vi "Switch Box Signal Select Control.vi"(0 "PhyChls":tag="Dev1/port0/line1:2", 1 "line grouping":i32(ring) items=["one channel for each line", "one channel for all lines"], 2 "Signal":T1(ring), 5 "All OFF":bool, 7 "Dout Inv":bool[](array[boolean])=[FALSE, FALSE], 11 "ErrIn":errorcluster, 12 "SimOn":bool, 13 "Init":bool, 14 "Stop":bool) -> (15 "ErrOut":errorcluster)   [LabVIEW 2013]
uses:
  <vilib>/DAQmx/write.llb/DAQmx Write (Digital 1D Bool NChan 1Samp 1Line).vi
  <vilib>/DAQmx/create/channels.llb/DAQmx Create Channel (DO-Digital Output).vi
  <vilib>/DAQmx/miscellaneous.llb/DAQmx Fill In Error Info.vi
panel:
  # "ER2007"
  # "SCL1 -> SCL2"
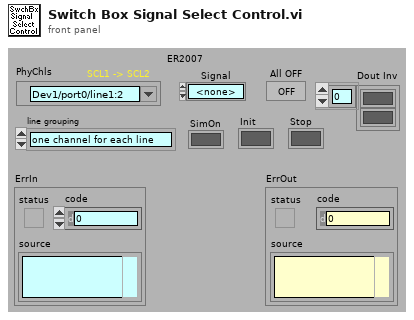
[diagram p1: front panel]
types:
  T1 = enum16{"<none>", "Signal 1", "Signal 2", "Signal 3"}
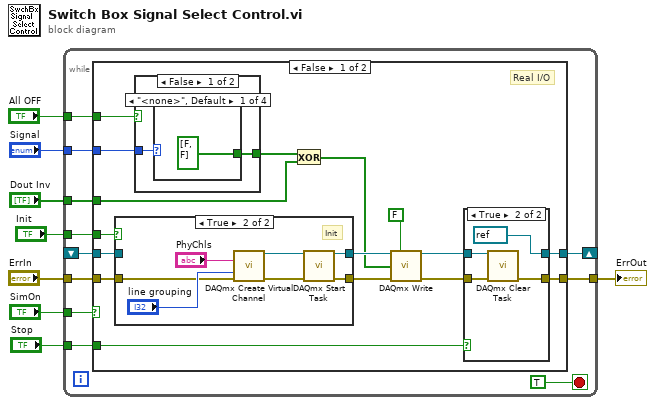
[diagram p0: block diagram]
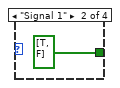
[diagram p4: hidden frame]
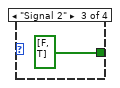
[diagram p5: hidden frame]
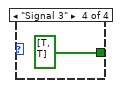
[diagram p6: hidden frame]
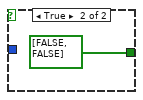
[diagram p7: hidden frame]
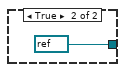
[diagram p9: hidden frame]
diagram:
  n1 = while {
    tunnel: "ErrIn" -> [w19]
    tunnel: [w18] -> w7
    tunnel: "SimOn" -> [w17]
    tunnel: "Stop" -> [w16]
    tunnel: "All OFF" -> [w15]
    tunnel: "Signal" -> [w14]
    tunnel: "Dout Inv" -> [w13]
    shift-right: [w12] -> _
    shift-left: _ -> [w10]
    tunnel: "Init" -> [w9]
    stop <- TRUE stop-if-true
    n2 = case shown="False" w17 {
      tunnel: w19 -> [w35 w61]
      tunnel: [w29 w61] -> w18
      tunnel: w16 -> [w26 _]
      tunnel: w15 -> [w25 _]
      tunnel: w14 -> [w24 _]
      tunnel: w13 -> [w23 _]
      tunnel: [w22 w58] -> w12
      tunnel: w10 -> [w21 w60]
      tunnel: w9 -> [w20 w59]
      frame False {
        # "Real I/O"
        n3 = case shown="True" w20 {
          tunnel: w35 -> [w42 w48]
          tunnel: [w42 w46] -> w34
          tunnel: [w43 w44] -> w33
          tunnel: w21 -> [w43 _]
          frame False {
          }
          frame True {
            # "Init"
            n4 = call-poly <vilib>:"DAQmx Create Virtual Channel.vi"("lines"="PhyChls", "line grouping"="line grouping", "error in"=w48) -> ("task out"=w45:refnum<k21>, "error out"=w47:errorcluster)  [unwired: 11 in]
            n5 = call <vilib>:"DAQmx Start Task.vi"("task/channels in"=w45, "error in"=w47) -> ("task out"=w44:refnum<k21>, "error out"=w46:errorcluster)  [unwired: 12 in]
          }
        }
        n6 = case shown="False" w25 {
          tunnel: [w51 bool[] [FALSE, FALSE]] -> w28
          tunnel: w24 -> [w52 _]
          frame False {
            n7 = case shown="\"<none>\", Default" w52 {
              tunnel: [bool[] [FALSE, FALSE] bool[] [TRUE, FALSE] bool[] [FALSE, TRUE] bool[] [TRUE, TRUE]] -> w51
              frame "<none>", Default {
              }
              frame "Signal 1" {
              }
              frame "Signal 2" {
              }
              frame "Signal 3" {
              }
            }
          }
          frame True {
          }
        }
        n8 = Exclusive Or(1:w23, 2:w28) -> (0:w27:bool[])
        n9 = call-poly <vilib>:"DAQmx Write.vi"("task/channels in"=w33, "auto start"=FALSE, "data"=w27, "error in"=w34) -> ("task out"=w30:refnum<k21>, "error out"=w31:errorcluster)  [unwired: 9 in, 1 out]
        n10 = case shown="True" w26 {
          tunnel: w31 -> [w36 w41]
          tunnel: w30 -> [w37 w40]
          tunnel: [w36 w39] -> w29
          tunnel: [w37 refnum<k21> refnum ("task out")] -> w22
          frame False {
          }
          frame True {
            n11 = call <vilib>:"DAQmx Clear Task.vi"("task in"=w40, "error in"=w41) -> ("error out"=w39:errorcluster)  [unwired: 13 in]
          }
        }
      }
      frame True {
        # "Simulation"
        n12 = case shown="False" w59 {
          tunnel: w60 -> [w62 _]
          tunnel: [w62 refnum<k21> refnum ("task out")] -> w58
          frame False {
          }
          frame True {
          }
        }
      }
    }
  }
  "ErrOut" <- w7
